vi "GetUTCOffset.vi"(1 "Time":timestamp) -> (0 "UTC Offset (In Seconds)":dbl)   [LabVIEW 2015]
panel:
  out "x/y":dbl
  out "current time":timestamp
  out "Array":dbl[](array[numeric])
  in  "7/1/2000 (Local)":T1
  in  "1/1/2000 (Local)":T1
  # "Return the Offset from GMT for the given Time\n(Given time is displayed in local time)"
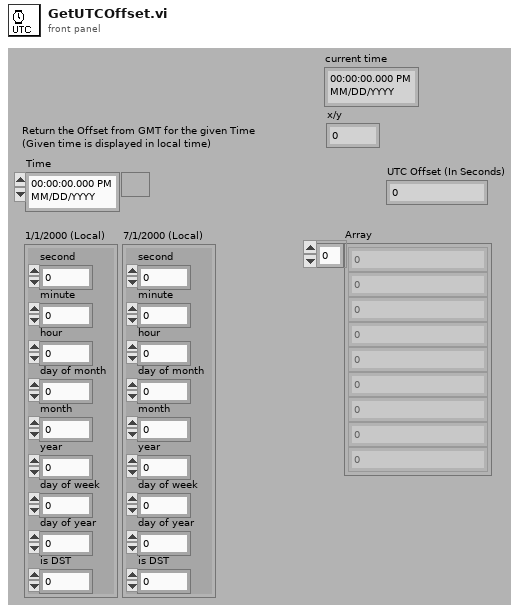
[diagram p1: front panel]
types:
  T1 = cluster{"second":i32, "minute":i32, "hour":i32, "day of month":i32, "month":i32, "year":i32, "day of week":i32, "day of year":i32, "is DST":i32}
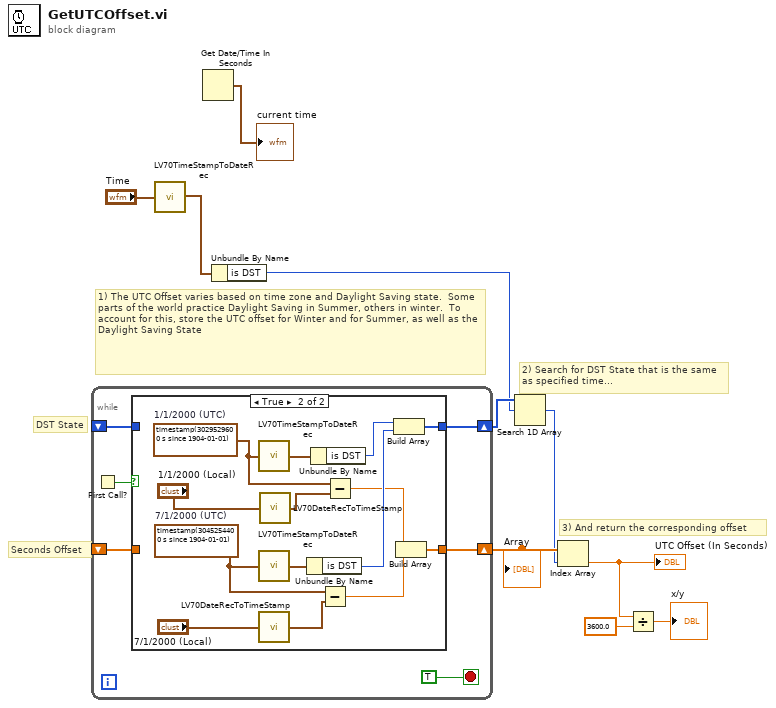
[diagram p0: block diagram]
diagram:
  # "3) And return the corresponding offset"
  # "2) Search for DST State that is the same\nas specified time..."
  # "Seconds Offset"
  # "DST State"
  # "1) The UTC Offset varies based on time zone and Daylight Saving state.  Some parts of the world practice Daylight Saving in Summer, others in winter.  To account for this, store the UTC offset for Winter and for Summer, as well as the Daylight Saving State"
  n1 = while {
    shift-right: [w14] -> w9
    shift-left: _ -> [w13]
    shift-right: [w15] -> w7
    shift-left: _ -> [w12]
    stop <- TRUE stop-if-true
    n2 = First Call?() -> (First Call?: T/F=w11:bool)
    n3 = case shown="True" w11 {
      tunnel: [w17 w28] -> w15
      tunnel: [w18 w27] -> w14
      tunnel: w13 -> [w18 _]
      tunnel: w12 -> [w17 _]
      frame False {
      }
      frame True {
        w22 = timestamp(3045254400 s since 1904-01-01)  # 7/1/2000 (UTC)
        w24 = timestamp(3029529600 s since 1904-01-01)  # 1/1/2000 (UTC)
        n4 = call <vilib>:"LV70TimeStampToDateRec.vi"("time stamp"=w24) -> ("date time rec"=w32:T1)
        n5 = call <vilib>:"LV70TimeStampToDateRec.vi"("time stamp"=w22) -> ("date time rec"=w31:T1)
        n6 = call <vilib>:"LV70DateRecToTimeStamp.vi"("date time rec"="7/1/2000 (Local)") -> ("Time Stamp"=w21:timestamp)
        n7 = call <vilib>:"LV70DateRecToTimeStamp.vi"("date time rec"="1/1/2000 (Local)") -> ("Time Stamp"=w23:timestamp)
        n8 = Unbundle By Name(w31) -> ("is DST"=w29:i32)
        n9 = Unbundle By Name(w32) -> ("is DST"=w30:i32)
        n10 = Subtract(x=w22, y=w21) -> (x-y=w19:dbl)
        n11 = Subtract(x=w24, y=w23) -> (x-y=w20:dbl)
        n12 = Build Array(w30, w29) -> (w27:i32[])
        n13 = Build Array(w20, w19) -> (w28:dbl[])
      }
    }
  }
  "Array" <- w7
  n14 = call <vilib>:"LV70TimeStampToDateRec.vi"("time stamp"="Time") -> ("date time rec"=w10:T1)
  n15 = Get Date/Time In Seconds() -> (seconds since 1Jan1904=→"current time":timestamp)
  n16 = Unbundle By Name(w10) -> ("is DST"=w8:i32)
  n17 = Search 1D Array(1D array=w9, element=w8) -> (index of element=w6:i32)  [unwired: 1 in]
  n18 = Index Array(array=w7, index=w6) -> (element=w4:dbl)
  "UTC Offset (In Seconds)" <- w4
  n19 = Divide(x=w4, y=3600.0) -> (x/y=→"x/y":dbl)
